vi "test Quadrature.vi"(8 "error in (no error)":errorcluster, 11 "TestCase in":refnum<class "Scan Engine Specialty Digital System Tests.lvclass">) -> (0 "error out":errorcluster, 3 "TestCase out":refnum<class "Scan Engine Specialty Digital System Tests.lvclass">)   [LabVIEW 2019, in "Scan Engine Specialty Digital System Tests.lvclass"]
uses:
  Scan Engine Specialty Digital System Tests.lvclass
  C:/Users/nitest/Desktop/Git 2019/niveristand-custom-device-testing-tools/VeriStandTestCase/VeriStandTestCase.lvclass
  <vilib>/NI VeriStand/Execution/Workspace/NI VeriStand - Get Single Channel Value.vi
  <vilib>/addons/_JKI Toolkits/VI Tester/TestCase.llb/TestCase.lvclass
  <vilib>/NI VeriStand/Execution/Workspace/NI_VS Workspace ExecutionAPI.lvlib
  C:/Program Files (x86)/National Instruments/LabVIEW 2019/vi.lib/addons/_JKI Toolkits/VI Tester/TestCase.llb/TestCase.lvclass
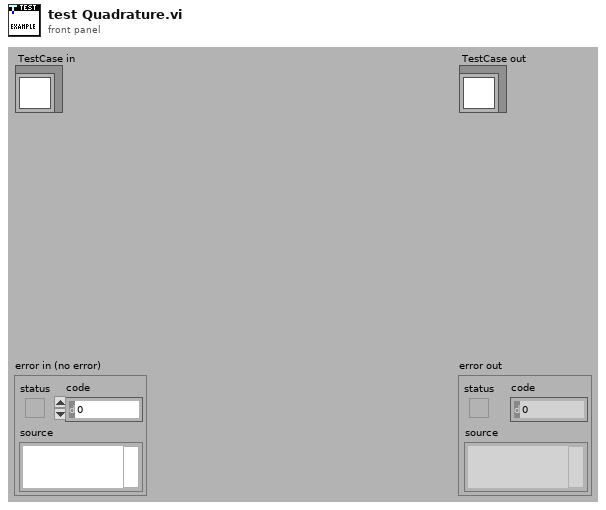
[diagram p1: front panel]
types:
  T1 = typedef "NI_VS Workspace ExecutionAPI.lvlib/WorkspaceAPI.ctl" = refnum<k24>
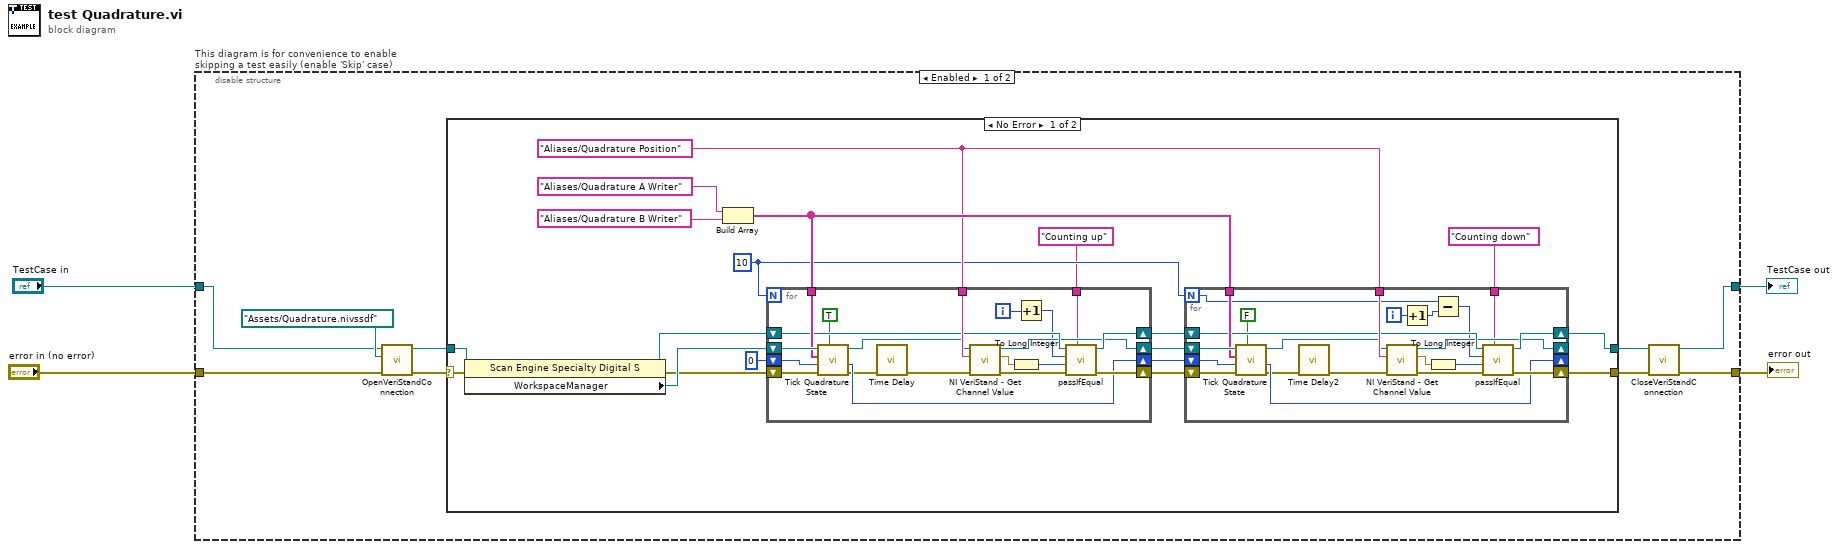
[diagram p0: block diagram]
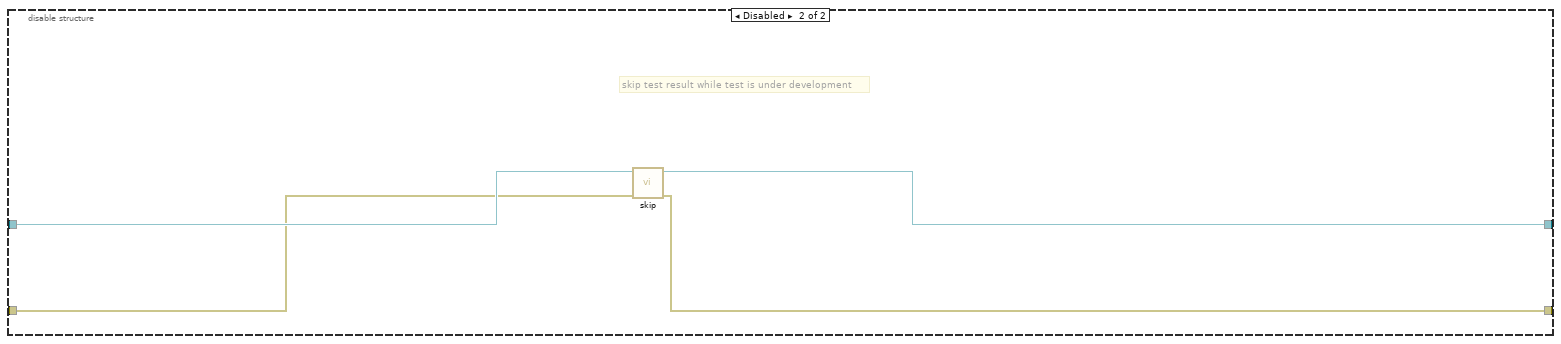
[diagram p3: hidden frame]
diagram:
  n1 = disable-structure "This diagram is for convenience to enable skipping a test easily (enable 'Skip' case)" shown="Enabled" {
    disable-tunnel: "TestCase in" -> [w9 w80]
    disable-tunnel: [w6 w78] -> w1
    disable-tunnel: [w7 w79] -> w3
    disable-tunnel: "error in (no error)" -> [w11 w77]
    frame Enabled {
      n2 = call-dynamic "OpenVeriStandConnection.vi"("error in (no error)"=w11, "System Definition File"=path "Assets/Quadrature.nivssdf", "VeriStand Test Case in"=w9) -> ("error out"=w12:errorcluster, "VeriStand Test Case out"=w10:refnum<class "Scan Engine Specialty Digital System Tests.lvclass">)  [unwired: 6 in, 1 out]
      n3 = case shown="No Error" w12 {
        selector: w12 -> [w32 w76]
        tunnel: [w17 w76] -> w8
        tunnel: [w16 w75] -> w5
        tunnel: w10 -> [w31 w75]
        frame No Error {
          w20 = 10
          w23 = "Aliases/Quadrature Position" ("Channel")
          n4 = property class="Scan Engine Specialty Digital S"(reference=w31, error in=w32) -> (reference out=w26:refnum<class "Scan Engine Specialty Digital System Tests.lvclass">, error out=w29:errorcluster, "WorkspaceManager"=w30:T1)
          n5 = Build Array("Aliases/Quadrature A Writer" ("Channel"), "Aliases/Quadrature B Writer" ("Channel")) -> (w24:string[])
          n6 = for {
            N: w20 -> [_]
            tunnel: w23 -> [w74]
            tunnel: w24 -> [w66]
            shift-right: [w72] -> w21
            shift-left: w29 -> [w67]
            shift-right: [w71] -> w22
            shift-left: w26 -> [w65]
            shift-right: [w63] -> w19
            shift-left: 0 ("New State") -> [w64]
            shift-right: [w62] -> w18
            shift-left: w30 -> [w68]
            tunnel: "Counting up" ("Channel") -> [w55]
            i -> [w60]
            n7 = call "Tick Quadrature State.vi"("Forward? (T)"=TRUE, "error in (no error)"=w67, "Current State"=w64, "Channels"=w66, "WorkspaceManager in"=w68) -> ("error out"=w56:errorcluster, "New State"=w63:i32, "WorkspaceManager out"=w69:T1)  [unwired: 4 in]
            n8 = call "Time Delay"("error in (no error)"=w56) -> ("error out"=w57:errorcluster)  [unwired: 10 in]
            n9 = call-poly <vilib>:"NI VeriStand - Get Channel Value.vi"("error in (no error)"=w57, "Channel"=w74, "WorkspaceManager in"=w69) -> ("error out"=w73:errorcluster, "Value"=w70:dbl, "WorkspaceManager out"=w62:T1)  [unwired: 6 in]
            n10 = To Long Integer(number=w70) -> (32bit integer=w59:i32)
            n11 = Increment(x=w60) -> (x+1=w58:i32)
            n12 = call-dynamic "passIfEqual.vi"("custom report message (\"\")"=w55, "error in (no error)"=w73, "y"=w59, "x"=w58, "TestCase in"=w65) -> ("error out"=w72:errorcluster, "TestCase out"=w71:refnum<class "Scan Engine Specialty Digital System Tests.lvclass">)  [unwired: 5 in]
          }
          n13 = for {
            N: w20 -> [w39]
            tunnel: w23 -> [w54]
            tunnel: w24 -> [w46]
            shift-right: [w52] -> w17
            shift-left: w21 -> [w47]
            shift-right: [w51] -> w16
            shift-left: w22 -> [w45]
            shift-right: [w43] -> _
            shift-left: w19 -> [w44]
            shift-right: [w42] -> _
            shift-left: w18 -> [w48]
            tunnel: "Counting down" ("Channel") -> [w33]
            i -> [w38]
            n14 = call "Tick Quadrature State.vi"("Forward? (T)"=FALSE, "error in (no error)"=w47, "Current State"=w44, "Channels"=w46, "WorkspaceManager in"=w48) -> ("error out"=w35:errorcluster, "New State"=w43:i32, "WorkspaceManager out"=w49:T1)  [unwired: 4 in]
            n15 = call "Time Delay2"("error in (no error)"=w35) -> ("error out"=w34:errorcluster)  [unwired: 10 in]
            n16 = call-poly <vilib>:"NI VeriStand - Get Channel Value.vi"("error in (no error)"=w34, "Channel"=w54, "WorkspaceManager in"=w49) -> ("error out"=w53:errorcluster, "Value"=w50:dbl, "WorkspaceManager out"=w42:T1)  [unwired: 6 in]
            n17 = Increment(x=w38) -> (x+1=w37:i32)
            n18 = To Long Integer(number=w50) -> (32bit integer=w40:i32)
            n19 = Subtract(x=w39, y=w37) -> (x-y=w36:i32)
            n20 = call-dynamic "passIfEqual.vi"("custom report message (\"\")"=w33, "error in (no error)"=w53, "y"=w40, "x"=w36, "TestCase in"=w45) -> ("error out"=w52:errorcluster, "TestCase out"=w51:refnum<class "Scan Engine Specialty Digital System Tests.lvclass">)  [unwired: 5 in]
          }
        }
        frame Error {
        }
      }
      n21 = call-dynamic "CloseVeriStandConnection.vi"("error in (no error)"=w8, "VeriStand Test Case in"=w5) -> ("error out"=w7:errorcluster, "VeriStand Test Case out"=w6:refnum<class "Scan Engine Specialty Digital System Tests.lvclass">)  [unwired: 8 in]
    }
    frame Disabled {
      # "skip test result while test is under development"
      n22 = call <vilib>:"skip.vi"("error in (no error)"=w77, "TestCase in"=w80) -> ("error out"=w79:errorcluster, "TestCase out"=w78:refnum<class "Scan Engine Specialty Digital System Tests.lvclass">)  [unwired: 8 in]
    }
  }
  "error out" <- w3
  "TestCase out" <- w1
